vi "Unit To String.vi"(1 "Unit":T1) -> (0 "String":string)   [LabVIEW 2023, in "NI_HFNetworkAnalysis.lvlib"]
doc: "Transforms specified unit into a string."
uses:
  NI_HFNetworkAnalysis.lvlib
  Controls/Unit.ctl
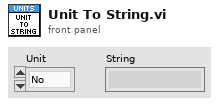
[diagram p1: front panel]
types:
  T1 = typedef "NI_HFNetworkAnalysis.lvlib/Unit.ctl" = enum16{"No", "s", "Hz", "V", "A", "Ohm", "W", "dB", "dBV", "dBA", "dBm", "percent", "rad", "deg"}
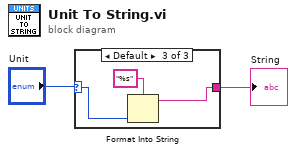
[diagram p0: block diagram]
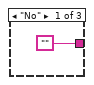
[diagram p2: hidden frame]
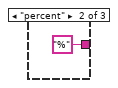
[diagram p3: hidden frame]
diagram:
  n1 = case shown="Default" "Unit" {
    selector: "Unit" -> [_ _ w6]
    tunnel: ["" "%" w5] -> w1
    frame "No" {
    }
    frame "percent" {
    }
    frame Default {
      n2 = Format Into String(format string="%s", w6) -> (resulting string=w5:string)  [unwired: 2 in, 1 out]
    }
  }
  "String" <- w1
